vi "decode fixed64.vi"(10 "read index in":i32, 11 "byte array in":u8[](array[numeric]) format="%.0b") -> (1 "u64":u64, 2 "read index out":i32)   [LabVIEW 2013, in "protocol buffers encoder.lvlib"]
uses:
  protocol buffers encoder.lvlib
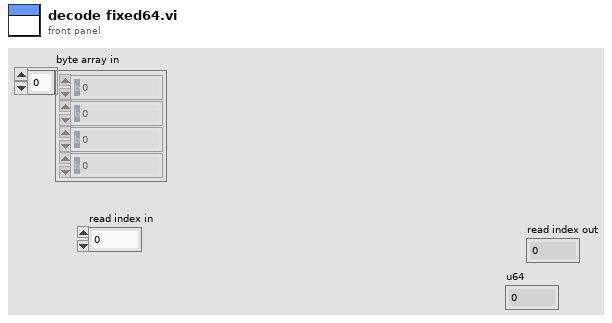
[diagram p1: front panel]
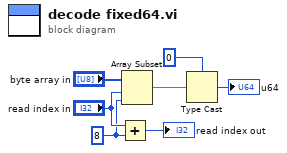
[diagram p0: block diagram]
diagram:
  w3 = 8 ("index")
  n1 = Add(x="read index in", y=w3) -> (x+y=→"read index out":i32)
  n2 = Array Subset(array="byte array in", index="read index in", length=w3) -> (w1:u8[])
  n3 = Type Cast(type=u64 0, x=w1) -> (*(type *) &x=→"u64":u64)
